vi "create client.vi"(8 "error in":errorcluster) -> (0 "error out":errorcluster, 3 "lvlibretls client socket out":refnum<class "lvlibretls client socket.lvclass">)   [LabVIEW 2016, in "lvlibretls client socket.lvclass"]
doc: "Creates a client object, which includes a parent configuration context. Libtls doesn't use a long-running client context, the 'client' context is only created when the connection is made."
uses:
  lvlibretls client socket.lvclass
  C:/Users/IEUser/Desktop/tlssimple/lvlibtls/context parent/lvlibretls configurable context.lvclass
  context parent/lvlibretls configurable context.lvclass
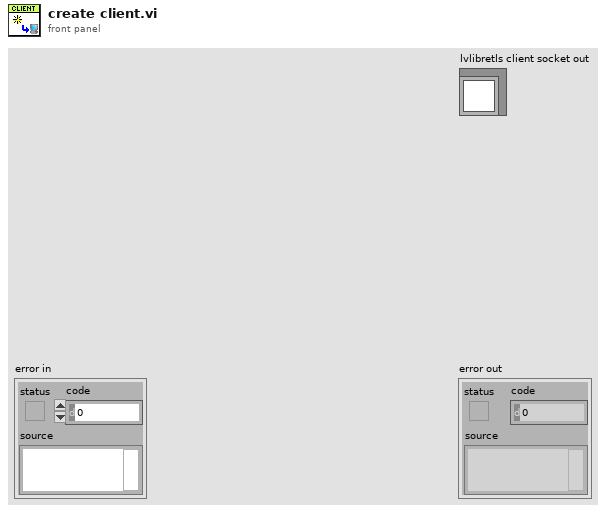
[diagram p1: front panel]
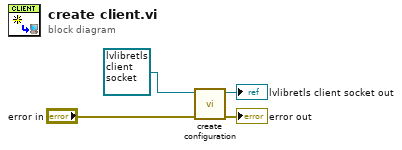
[diagram p0: block diagram]
diagram:
  n1 = call "create configuration.vi"("error in"="error in", "lvlibretls configurable context in"=refnum<class "lvlibretls client socket.lvclass"> refnum ("lvlibretls client socket in")) -> ("error out"=→"error out":errorcluster, "lvlibretls configurable context out"=→"lvlibretls client socket out":refnum<class "lvlibretls client socket.lvclass">)  [unwired: 8 in]
